vi "Switch tables test2.vi"() -> ()   [LabVIEW 2016]
uses:
  LV-Data/src/LV-Data.PG/LV-Data.PGSQL.lvclass
  <vilib>/addons/_JKI Toolkits/Caraya/classes/Test/Test.lvclass
  <vilib>/addons/_JKI Toolkits/Caraya/classes/Assert/Assert.lvclass
  <vilib>/addons/_JKI Toolkits/Caraya/classes/Assert/Assert Not Error.vi
panel:
  out "error out":errorcluster
  in  "error in (no error)":errorcluster
  out "Data.PG out":refnum<class "LV-Data.PGSQL.lvclass">
  in  "Data.PG":refnum<class "LV-Data.PGSQL.lvclass">
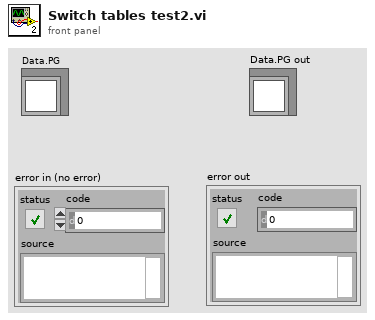
[diagram p1: front panel]
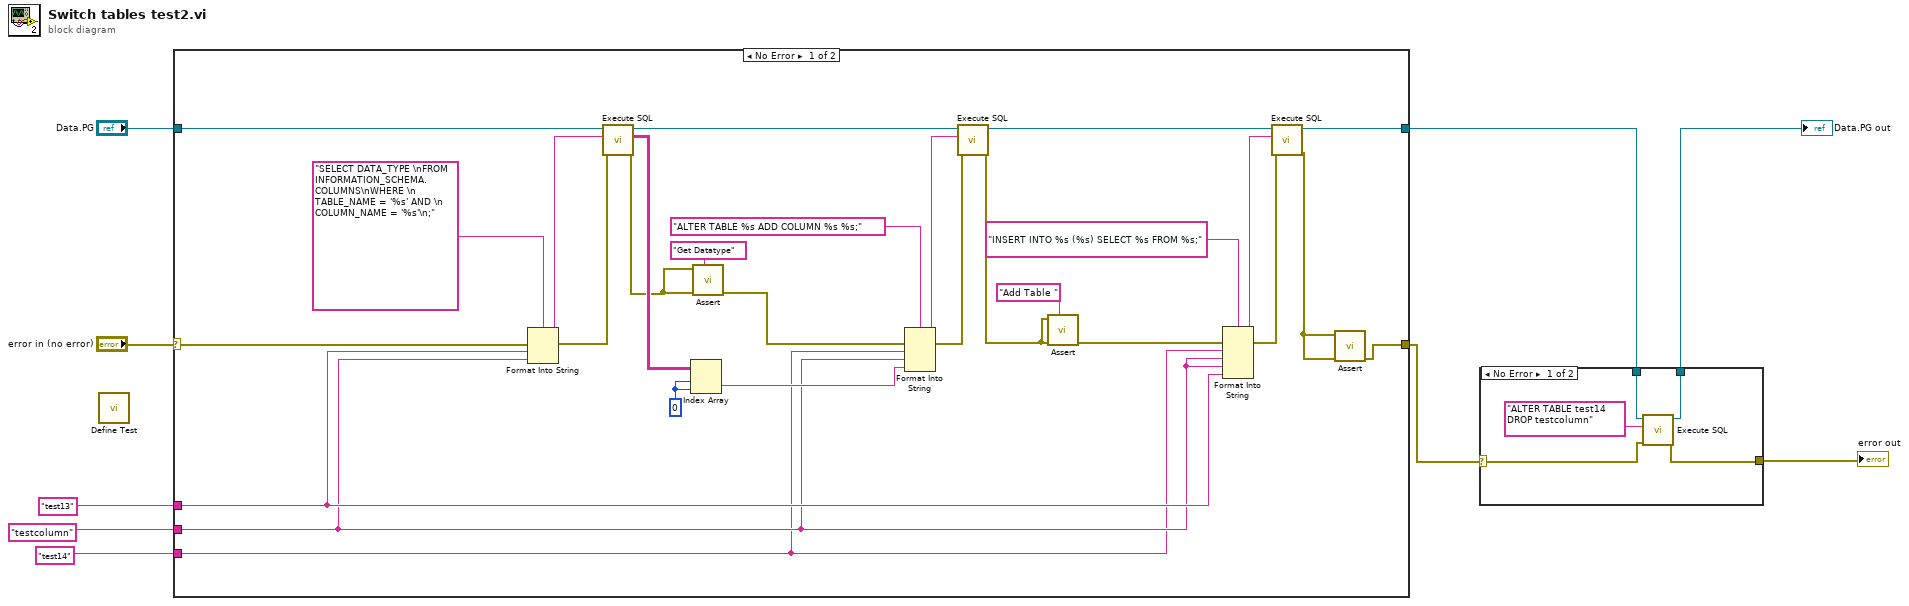
[diagram p0: block diagram]
diagram:
  n1 = call <vilib>:"Define Test.vi"() -> ()  [unwired: 11 in, 1 out]
  n2 = case shown="No Error" "error in (no error)" {
    selector: "error in (no error)" -> [w18 w38]
    tunnel: "test14" ("Old Column") -> [w20 _]
    tunnel: "testcolumn" ("Old Column") -> [w21 _]
    tunnel: "Data.PG" -> [w19 w39]
    tunnel: [w37 w39] -> w2
    tunnel: "test13" ("Old Table") -> [w23 _]
    tunnel: [w10 w38] -> w1
    frame No Error {
      w30 = 0 ("index (row)")
      n3 = Format Into String(format string="SELECT DATA_TYPE \nFROM INFORMATION_SCHEMA.COLUMNS\nWHERE \n     TABLE_NAME = '%s' AND \n     COLUMN_NAME = '%s'\n;", error in=w18, w23, w21) -> (resulting string=w25:string, error out=w28:errorcluster)  [unwired: 1 in]
      n4 = call "Execute SQL.vi"("error in"=w28, "SQL"=w25, "Data.PG"=w19) -> ("error out"=w16:errorcluster, "Result"=w36:string[][], "Data.PG out"=w32:refnum<class "LV-Data.PGSQL.lvclass">)  [unwired: 6 in]
      n5 = Index Array(array=w36, index (row)=w30, index (col)=w30) -> (element=w22:string)
      n6 = call-poly <vilib>:"Assert.vi"("Label"="Get Datatype", "error in (no error)"=w16, "Not Error?"=w16) -> ("error out"=w17:errorcluster)  [unwired: 8 in]
      n7 = Format Into String(format string="ALTER TABLE %s ADD COLUMN %s %s;", error in=w17, w20, w21, w22) -> (resulting string=w33:string, error out=w27:errorcluster)  [unwired: 1 in]
      n8 = call "Execute SQL.vi"("error in"=w27, "SQL"=w33, "Data.PG"=w32) -> ("error out"=w13:errorcluster, "Data.PG out"=w31:refnum<class "LV-Data.PGSQL.lvclass">)  [unwired: 6 in, 1 out]
      n9 = call-poly <vilib>:"Assert.vi"("Label"="Add Table ", "error in (no error)"=w13, "Not Error?"=w13) -> ("error out"=w14:errorcluster)  [unwired: 8 in]
      n10 = Format Into String(format string="INSERT INTO %s (%s) SELECT %s FROM %s;", error in=w14, w20, w21, w21, w23) -> (resulting string=w26:string, error out=w24:errorcluster)  [unwired: 1 in]
      n11 = call "Execute SQL.vi"("error in"=w24, "SQL"=w26, "Data.PG"=w31) -> ("error out"=w11:errorcluster, "Data.PG out"=w37:refnum<class "LV-Data.PGSQL.lvclass">)  [unwired: 6 in, 1 out]
      n12 = call-poly <vilib>:"Assert.vi"("error in (no error)"=w11, "Not Error?"=w11) -> ("error out"=w10:errorcluster)  [unwired: 9 in]
    }
    frame Error {
    }
  }
  n13 = case shown="No Error" w1 {
    selector: w1 -> [w43 w46]
    tunnel: [w42 w46] -> w4
    tunnel: [w44 w45] -> w3
    tunnel: w2 -> [w40 w45]
    frame No Error {
      n14 = call "Execute SQL.vi"("error in"=w43, "SQL"="ALTER TABLE test14 DROP testcolumn", "Data.PG"=w40) -> ("error out"=w42:errorcluster, "Data.PG out"=w44:refnum<class "LV-Data.PGSQL.lvclass">)  [unwired: 6 in, 1 out]
    }
    frame Error {
    }
  }
  "Data.PG out" <- w3
  "error out" <- w4
